vi "plotter.vi"() -> ()   [LabVIEW 2023]
uses:
  <vilib>/Instr/_visa.llb/VISA Configure Serial Port (Instr).vi
panel:
  out "Waveform Chart":dbl(graph)
  in  "stop":bool
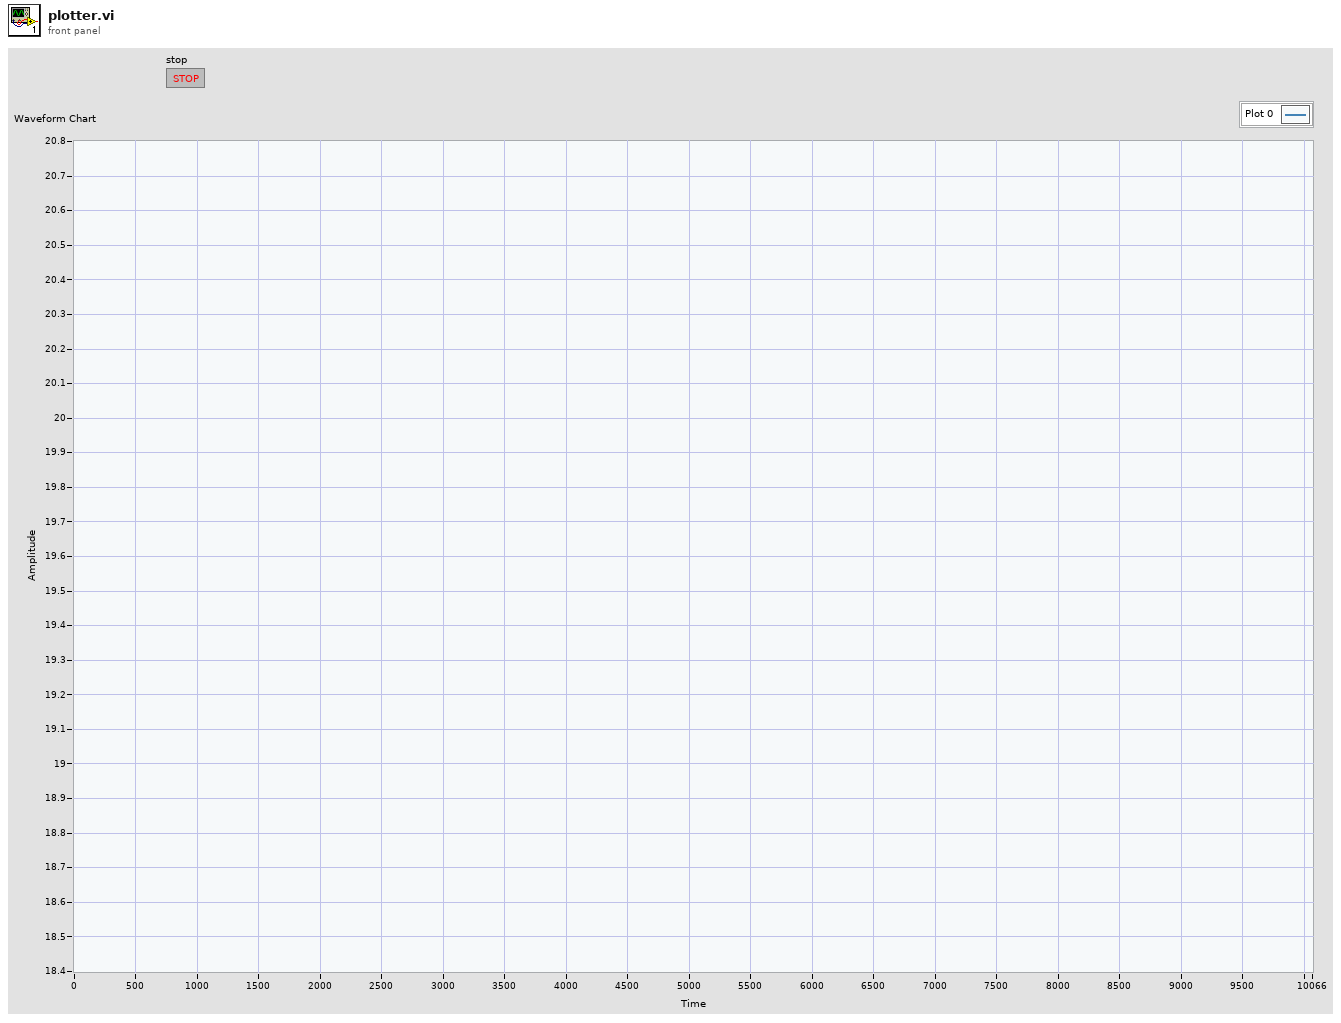
[diagram p1: front panel]
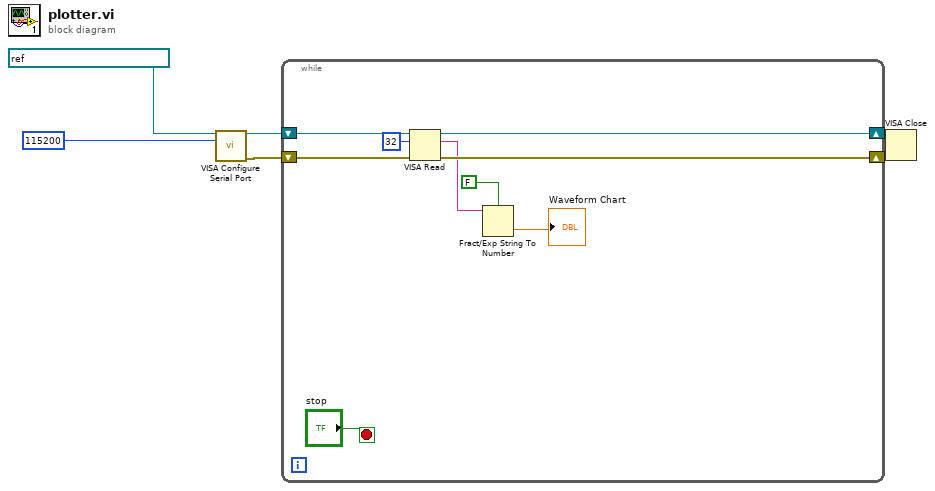
[diagram p0: block diagram]
diagram:
  n1 = call-poly "VISA Configure Serial Port"("VISA resource name"=refnum<visa-resource-name> "COM3", "baud rate (9600)"=u32 115200) -> ("VISA resource name out"=w4:refnum<visa-resource-name>, "error out"=w3:errorcluster)  [unwired: 12 in]
  n2 = while {
    shift-right: [w12] -> w2
    shift-left: w4 -> [w15]
    shift-right: [w11] -> w1
    shift-left: w3 -> [w14]
    stop <- "stop" stop-if-true
    n3 = VISA Read(VISA resource name=w15, byte count=u32 32, error in (no error)=w14) -> (VISA resource name out=w12:refnum<visa-resource-name>, read buffer=w9:string, error out=w11:errorcluster)  [unwired: 1 out]
    n4 = Fract/Exp String To Number(use system decimal point (T)=FALSE, string=w9) -> (number=→"Waveform Chart":dbl)  [unwired: 2 in, 1 out]
  }
  n5 = VISA Close(VISA resource name=w2, error in (no error)=w1) -> ()  [unwired: 1 out]
